vi "Generate Alarm Cleared Log Entry.vi"(11 "Alarm":T1) -> (3 "Log Entry":string)   [LabVIEW 2015, in "Alarm Handler Actor.lvclass"]
uses:
  Alarm Handler Actor.lvclass
  Active Alarm.ctl
  Alarm Details.ctl
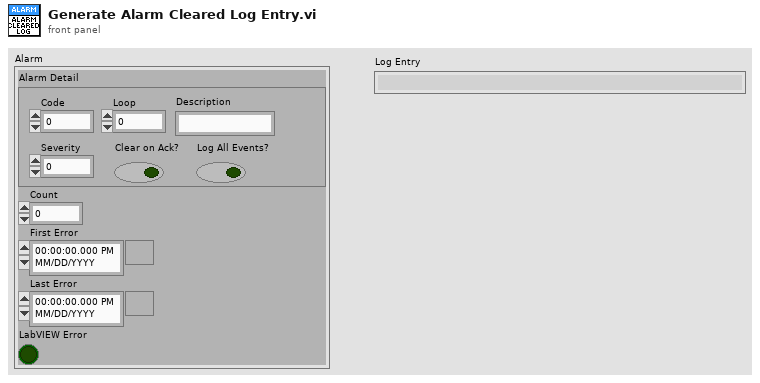
[diagram p1: front panel]
types:
  T1 = typedef "Alarm Handler Actor.lvclass/Active Alarm.ctl" = cluster{"Alarm Detail":T2, "Count":i32, "First Error":timestamp, "Last Error":timestamp, "LabVIEW Error":bool}
  T2 = typedef "Alarm Handler Actor.lvclass/Alarm Details.ctl" = cluster{"Code":i32, "Loop":i32, "Description":string, "Severity":i32, "Clear on Ack?":bool, "Log All Events?":bool}
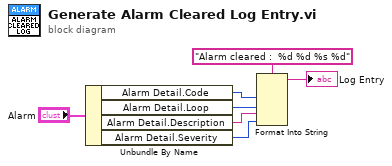
[diagram p0: block diagram]
diagram:
  n1 = Unbundle By Name("Alarm") -> ("Alarm Detail.Code"=w6:i32, "Alarm Detail.Loop"=w5:i32, "Alarm Detail.Description"=w4:string, "Alarm Detail.Severity"=w3:i32)
  n2 = Format Into String(format string="Alarm cleared :  %d %d %s %d", w6, w5, w4, w3) -> (resulting string=→"Log Entry":string)  [unwired: 2 in, 1 out]
